vi "Actor Core.vi"(8 "error in":errorcluster, 11 "Staff Manager UI in":refnum<class "Staff Manager UI.lvclass">) -> (0 "error out":errorcluster, 3 "Actor out":refnum<class "Actor.lvclass">)   [LabVIEW 2023, in "Staff Manager UI.lvlib" / "Staff Manager UI.lvclass"]
doc: "(<B>Filename</B>: Actor Framework.lvlib:Actor.lvclass:Actor Core.vi)\n\nReceives messages to the actor, reacts to them, and initiates any error handling that may shut the actor down.\n\nDescendant classes may override this VI to append parallel tasks for the actor to complete while it handles messages. Overrides use the Call Parent Class Method node."
uses:
  Staff Manager UI.lvclass
  C:/Users/bhaghyaraj/Trainings/NI Actor Framework/SDLC/UI Base/UI Base/UI Base.lvclass
  C:/Program Files/National Instruments/LabVIEW 2023/vi.lib/ActorFramework/Actor/Actor.lvclass
  <vilib>/ActorFramework/Actor/Actor.lvclass
  Staff Manager UI.lvclass/Staff Manager UI.ctl
  <vilib>/ActorFramework/Actor/Actor.lvclass/Actor.ctl
  <vilib>/ActorFramework/Message Enqueuer/Message Enqueuer.lvclass/Message Enqueuer.ctl
  <vilib>/ActorFramework/Message Enqueuer/Init from Existing Queue.vi
  <vilib>/ActorFramework/Message Enqueuer/Enqueue.vi
  <vilib>/ActorFramework/Stop Msg/Stop Msg.lvclass
  C:/Program Files/National Instruments/LabVIEW 2023/vi.lib/ActorFramework/Message/Message.lvclass
  <vilib>/ActorFramework/Message Priority Queue/Priority Enqueue.vi
  <vilib>/ActorFramework/Message Enqueuer/Message Enqueuer.lvclass
  UI Base/UI Base/UI Base.lvclass
panel:
  out "Staff Info":i32(listbox)
  # "Staff Management"
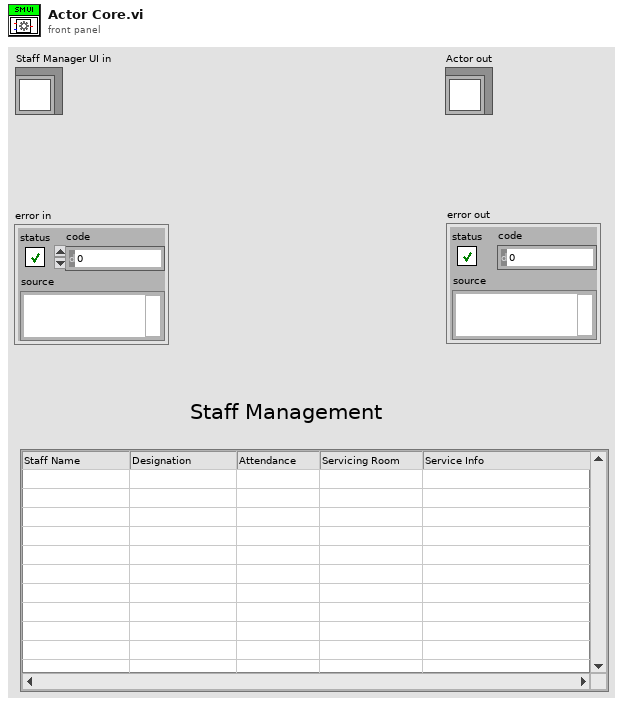
[diagram p1: front panel]
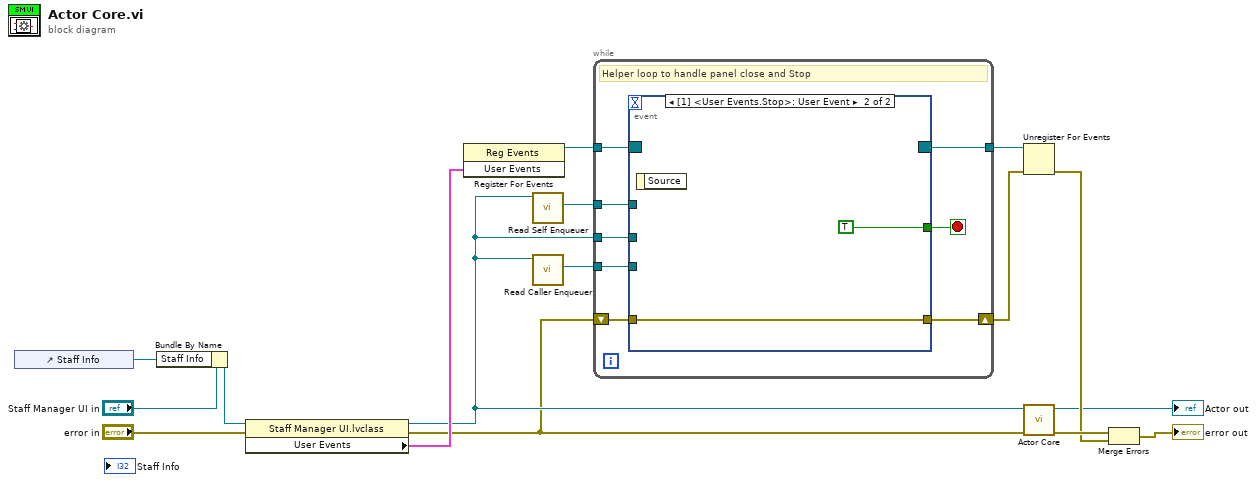
[diagram p0: block diagram]
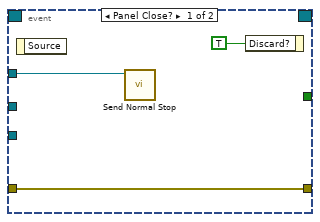
[diagram p2: hidden frame]
diagram:
  n1 = control-ref of="Staff Info"() -> (w1:refnum<vi>)
  n2 = Bundle By Name(cluster="Staff Manager UI in", "Staff Info"=w1) -> (w2:refnum<class "Staff Manager UI.lvclass">)
  n3 = property class="Staff Manager UI.lvclass"(reference=w2, error in="error in") -> (reference out=w9:refnum<class "Staff Manager UI.lvclass">, error out=w8:errorcluster, "User Events"=w12:cluster{"Stop":refnum<user-event>})
  n4 = register-events(w12) -> (reference out=w14:refnum<event-registration>)  [unwired: 2 in, 1 out]
  n5 = call <vilib>:"Read Self Enqueuer.vi"("Actor"=w9) -> ("Self Enqueuer"=w13:refnum<class "Message Enqueuer.lvclass">)  [unwired: 10 in]
  n6 = call <vilib>:"Read Caller Enqueuer.vi"("Actor"=w9) -> ("Caller Enqueuer"=w10:refnum<class "Message Enqueuer.lvclass">)  [unwired: 10 in]
  n7 = while {
    tunnel: w13 -> [w24]
    tunnel: w14 -> [w23]
    tunnel: [w21] -> w15
    tunnel: w10 -> [w20]
    tunnel: w9 -> [w19]
    shift-right: [w17] -> w7
    shift-left: w8 -> [w18]
    stop <- w22 stop-if-true
    # "Helper loop to handle panel close and Stop"
    n8 = event shown="[1] <User Events.Stop>: User Event" {
      selector: w23 -> [_ _]
      dyn-events: [_ _] -> w21
      timeout: _ -> [_ _]
      tunnel: w24 -> [w26 _]
      tunnel: [_ TRUE] -> w22
      tunnel: w20 -> [_ _]
      tunnel: w19 -> [_ _]
      tunnel: w18 -> [w25 w28]
      tunnel: [w25 w28] -> w17
      event Panel Close? {
        n9 = event-data() -> ()  [unwired: 1 in, 1 out]
        n10 = call <vilib>:"Send Normal Stop.vi"("Message Enqueuer"=w26) -> ()  [unwired: 10 in, 1 out]
        n11 = event-data("Discard?"=TRUE) -> ()  [unwired: 1 in, 1 out]
      }
      event User Event {
        n12 = event-data() -> ()  [unwired: 1 in, 1 out]
      }
    }
  }
  n13 = Unregister For Events(event registration refnum=w15, error in=w7) -> (error out=w11:errorcluster)
  n14 = call-parent "Actor Core.vi"("error in"=w8, "Actor in"=w9) -> ("error out"=w16:errorcluster, "Actor out"=→"Actor out":refnum<class "Actor.lvclass">)  [unwired: 8 in]
  n15 = Merge Errors(w16, w11) -> (→"error out":errorcluster)
